vi "Fault_Seq_Read.vi"(7 "Seq ERD In":T1[](array[typedef]) {"ERD Number" format="%.0x"}) -> (4 "Seq Buffer Status":T2, 8 "String":string)   [LabVIEW 2016]
uses:
  type defs/Fault_Buffer_Status.ctl
  Common/LabVIEW GEA2 Toolkit/LabVIEW_GEA2_Toolkit.lvlibp/type defs/ERD Read Data Out.ctl
  Common/LabVIEW GEA2 Toolkit/LabVIEW_GEA2_Toolkit.lvlibp
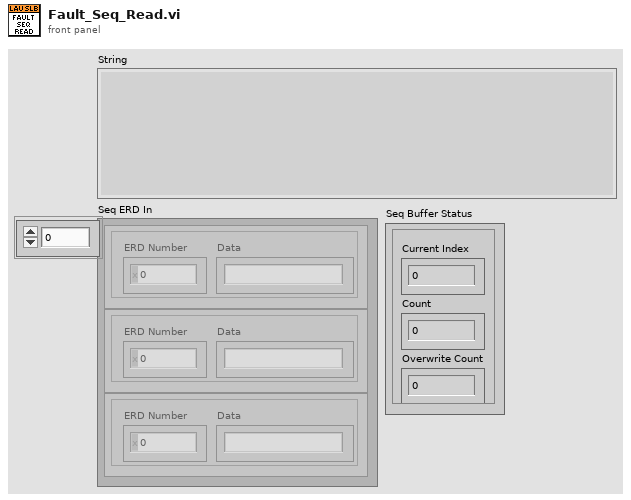
[diagram p1: front panel]
types:
  T1 = typedef "LabVIEW_GEA2_Toolkit.lvlibp/ERD Read Data Out.ctl" = cluster{"ERD Number":u16, "Data":string}
  T2 = typedef "Fault_Buffer_Status.ctl" = cluster{"Current Index":u16, "Count":u16, "Overwrite Count":u16}
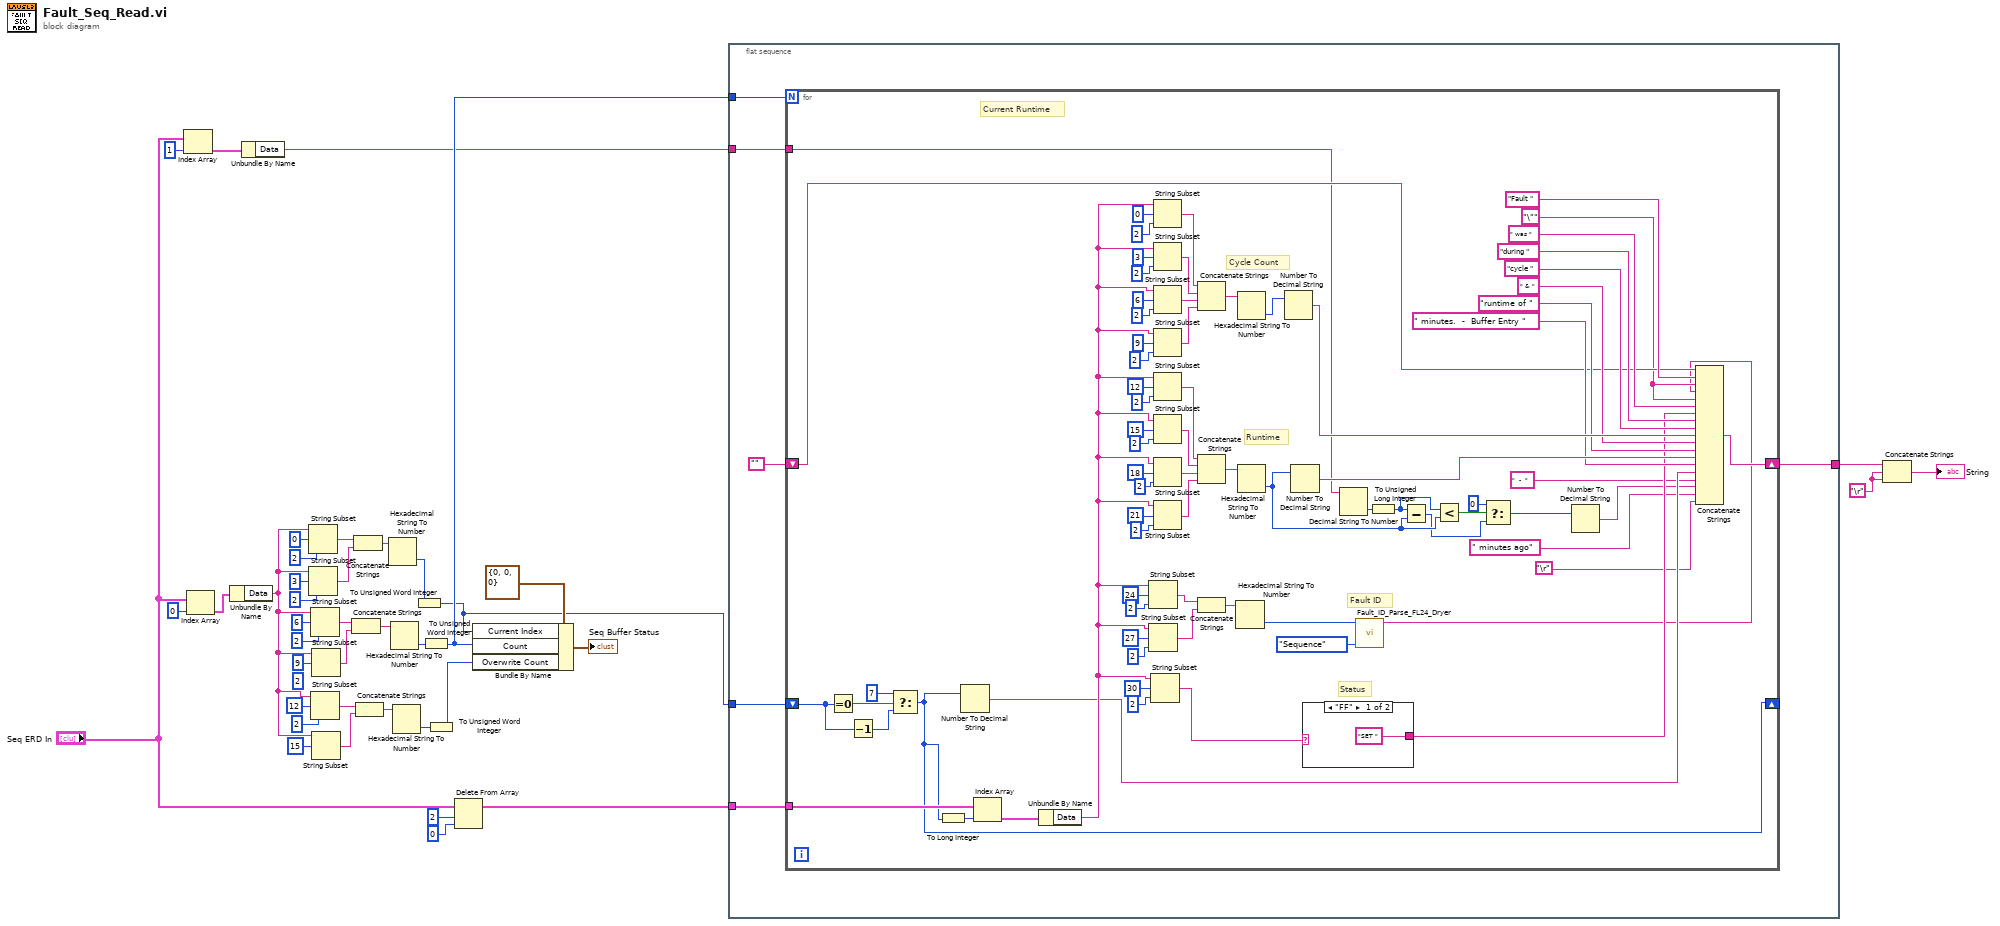
[diagram p0: block diagram]
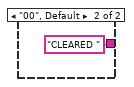
[diagram p2: hidden frame]
diagram:
  (unwired) 2 ("length (rest)")
  w39 = "\r"
  n1 = Index Array(array="Seq ERD In", index=1) -> (element=w6:T1)
  n2 = Index Array(array="Seq ERD In", index=0) -> (element=w37:T1)
  n3 = Unbundle By Name(w37) -> ("Data"=w26:string)
  n4 = Unbundle By Name(w6) -> ("Data"=w5:string)
  n5 = String Subset(string=w26, offset (0)=0, length (rest)=2 ("length (rest)")) -> (substring=w25:string)
  n6 = String Subset(string=w26, offset (0)=3, length (rest)=2 ("length (rest)")) -> (substring=w24:string)
  n7 = String Subset(string=w26, offset (0)=6, length (rest)=2 ("length (rest)")) -> (substring=w23:string)
  n8 = String Subset(string=w26, offset (0)=12, length (rest)=2 ("length (rest)")) -> (substring=w21:string)
  n9 = String Subset(string=w26, offset (0)=9) -> (substring=w22:string)  [unwired: 1 in]
  n10 = String Subset(string=w26, offset (0)=15) -> (substring=w20:string)  [unwired: 1 in]
  n11 = Concatenate Strings(w23, w22) -> (w18:string)
  n12 = Concatenate Strings(w25, w24) -> (w19:string)
  n13 = Concatenate Strings(w21, w20) -> (w17:string)
  n14 = Hexadecimal String To Number(string=w19) -> (number=w15:u32)  [unwired: 2 in, 1 out]
  n15 = Hexadecimal String To Number(string=w18) -> (number=w14:u32)  [unwired: 2 in, 1 out]
  n16 = Hexadecimal String To Number(string=w17) -> (number=w13:u32)  [unwired: 2 in, 1 out]
  n17 = To Unsigned Word Integer(number=w15) -> (unsigned 16bit integer=w9:u16)
  n18 = To Unsigned Word Integer(number=w14) -> (unsigned 16bit integer=w10:u16)
  n19 = To Unsigned Word Integer(number=w13) -> (unsigned 16bit integer=w11:u16)
  n20 = Delete From Array(array="Seq ERD In", length=2, index=0) -> (array with subset deleted=w2:T1[])  [unwired: 1 out]
  n21 = Bundle By Name(cluster=T2 {"Current Index"=0, "Count"=0, "Overwrite Count"=0} ("Buffer Status"), "Current Index"=w9, "Count"=w10, "Overwrite Count"=w11) -> (→"Seq Buffer Status":T2)
  n22 = flat-sequence {
    tunnel: w2 -> [w46]
    tunnel: w9 -> [w45]
    tunnel: [w44] -> w40
    tunnel: w10 -> [w42]
    tunnel: w5 -> [w41]
    frame #0 {
      n23 = for {
        N: w42 -> [_]
        tunnel: w46 -> [w116]
        shift-right: [w65] -> _
        shift-left: w45 -> [w120]
        shift-right: [w67] -> w44
        shift-left: "" -> [w66]
        tunnel: w41 -> [w49]
        w63 = "\"" ("string")
        # "Current Runtime"
        # "Status"
        # "Fault ID"
        # "Runtime"
        # "Cycle Count"
        n24 = Equal To 0?(x=w120) -> (x = 0?=w121:bool)
        n25 = Decrement(x=w120) -> (x-1=w119:u16)
        n26 = Select(t=u16 7, s=w121, f=w119) -> (s? t:f=w65:u16)
        n27 = To Long Integer(number=w65) -> (32bit integer=w117:i32)
        n28 = Number To Decimal String(number=w65) -> (decimal integer string=w64:string)  [unwired: 1 in]
        n29 = Index Array(array=w116, index=w117) -> (element=w115:T1)
        n30 = Unbundle By Name(w115) -> ("Data"=w78:string)
        n31 = String Subset(string=w78, offset (0)=24, length (rest)=2 ("length (rest)")) -> (substring=w94:string)
        n32 = String Subset(string=w78, offset (0)=27, length (rest)=2 ("length (rest)")) -> (substring=w93:string)
        n33 = String Subset(string=w78, offset (0)=30, length (rest)=2 ("length (rest)")) -> (substring=w79:string)
        n34 = String Subset(string=w78, offset (0)=0, length (rest)=2 ("length (rest)")) -> (substring=w110:string)
        n35 = String Subset(string=w78, offset (0)=3, length (rest)=2 ("length (rest)")) -> (substring=w109:string)
        n36 = String Subset(string=w78, offset (0)=6, length (rest)=2 ("length (rest)")) -> (substring=w108:string)
        n37 = String Subset(string=w78, offset (0)=9, length (rest)=2 ("length (rest)")) -> (substring=w107:string)
        n38 = String Subset(string=w78, offset (0)=12, length (rest)=2 ("length (rest)")) -> (substring=w101:string)
        n39 = String Subset(string=w78, offset (0)=15, length (rest)=2 ("length (rest)")) -> (substring=w102:string)
        n40 = String Subset(string=w78, offset (0)=18, length (rest)=2 ("length (rest)")) -> (substring=w103:string)
        n41 = String Subset(string=w78, offset (0)=21, length (rest)=2 ("length (rest)")) -> (substring=w104:string)
        n42 = Concatenate Strings(w110, w109, w108, w107) -> (w106:string)
        n43 = Concatenate Strings(w101, w102, w103, w104) -> (w105:string)
        n44 = Concatenate Strings(w94, w93) -> (w92:string)
        n45 = Hexadecimal String To Number(string=w92) -> (number=w56:u32)  [unwired: 2 in, 1 out]
        n46 = Hexadecimal String To Number(string=w106) -> (number=w77:u32)  [unwired: 2 in, 1 out]
        n47 = Hexadecimal String To Number(string=w105) -> (number=w52:u32)  [unwired: 2 in, 1 out]
        n48 = Number To Decimal String(number=w77) -> (decimal integer string=w72:string)  [unwired: 1 in]
        n49 = Number To Decimal String(number=w52) -> (decimal integer string=w69:string)  [unwired: 1 in]
        n50 = case shown="\"FF\"" w79 {
          tunnel: ["SET " "CLEARED "] -> w62
          frame "FF" {
          }
          frame "00", Default {
          }
        }
        n51 = Decimal String To Number(string=w49) -> (number=w58:i32)  [unwired: 2 in, 1 out]
        n52 = call "Fault_ID_Parse_FL24_Dryer.vi"("Enum"=enum16{"Sequence", "Table"}."Sequence", "Numeric"=w56) -> ("String"=w48:string)  [unwired: 9 in]
        n53 = To Unsigned Long Integer(number=w58) -> (unsigned 32bit integer=w53:u32)
        n54 = Subtract(x=w53, y=w52) -> (x-y=w51:u32)
        n55 = Less?(x=w53, y=w52) -> (x < y?=w54:bool)
        n56 = Select(t=u32 0, s=w54, f=w51) -> (s? t:f=w50:u32)
        n57 = Number To Decimal String(number=w50) -> (decimal integer string=w57:string)  [unwired: 1 in]
        n58 = Concatenate Strings(w66, "Fault " ("string"), w63, w48, w63, " was " ("string"), w62, "during " ("string"), "cycle " ("string"), w72, " & " ("string"), "runtime of " ("string"), w69, " minutes.  -  Buffer Entry " ("string"), w64, "  -  " ("string"), w57, " minutes ago" ("string"), "\r") -> (w67:string)
      }
    }
  }
  n59 = Concatenate Strings(w40, w39, w39) -> (→"String":string)
